vi "游标显示-快关试验.vi"(3 "计算参数 in":T2, 4 "试验模式":string, 5 "reference in":refnum<vi>) -> (0 "计算参数 out":T2, 2 "reference out":refnum<vi>)   [LabVIEW 2013]
panel:
  in  "Array":string[](array[string])=["行程", "电气", "油压1"]
  out "Yrange":dbl
  out "Xrange":dbl
  in  "Cursor":T1
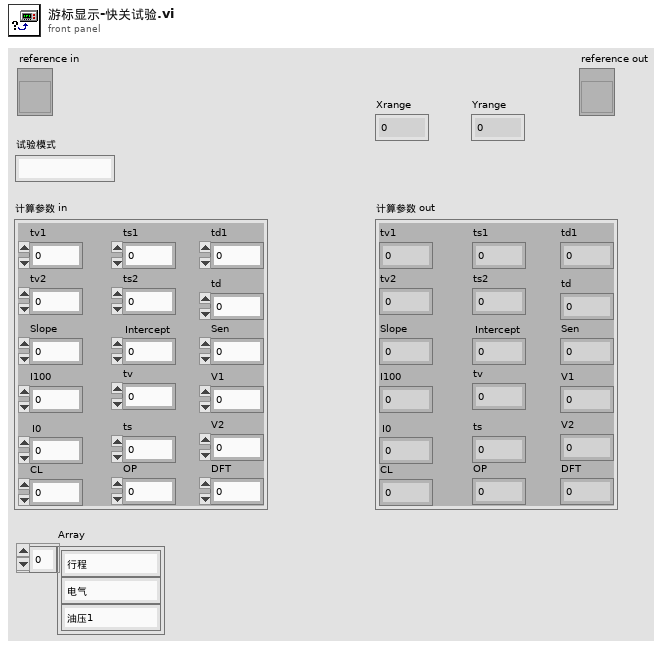
[diagram p1: front panel]
types:
  T1 = cluster{"Name":string, "Color":u32, "Style":u8, "Point Style":u8, "Name Visible":bool, "Allow Drag":bool, "Cursor Mode":u32, "Plot":i32, "Index":i32, "Position":cluster{"X":dbl, "Y":dbl}, "X Scale":u32, "Y Scale":u32, "Watch Plots":i32[], "Watch All Plots":bool, "Plot Area":i32, "Label Offset":cluster{"X":dbl, "Y":dbl}}
  T2 = cluster{"tv1":dbl, "tv2":dbl, "tv":dbl, "ts1":dbl, "ts2":dbl, "ts":dbl, "td1":dbl, "td":dbl, "Slope":dbl, "Intercept":dbl, "I100":dbl, "I0":dbl, "Sen":dbl, "V1":dbl, "V2":dbl, "CL":dbl, "OP":dbl, "DFT":dbl}
  T3 = cluster{"Name":string, "Color":u32, "Style":u8, "Point Style":u8, "Name Visible":bool, "Allow Drag":bool, "Cursor Mode":u32, "Plot":i32, "Index":i32, "Position":cluster{"X":dbl, "Y":dbl}, "X Scale":u32, "Y Scale":u32, "Watch Plots":i32[], "Watch All Plots":bool, "Plot Area":i32, "Label Offset":cluster{"X":dbl, "Y":dbl}}[]
  T4 = typedef "LVCursorListTypeDef.ctl" = cluster{"Name":string, "Color":u32, "Style":u8, "Point Style":u8, "Name Visible":bool, "Allow Drag":bool, "Cursor Mode":u32, "Plot":i32, "Index":i32, "Position":cluster{"X":dbl, "Y":dbl}, "X Scale":u32, "Y Scale":u32, "Watch Plots":i32[], "Watch All Plots":bool, "Plot Area":i32, "Label Offset":cluster{"X":dbl, "Y":dbl}}[]
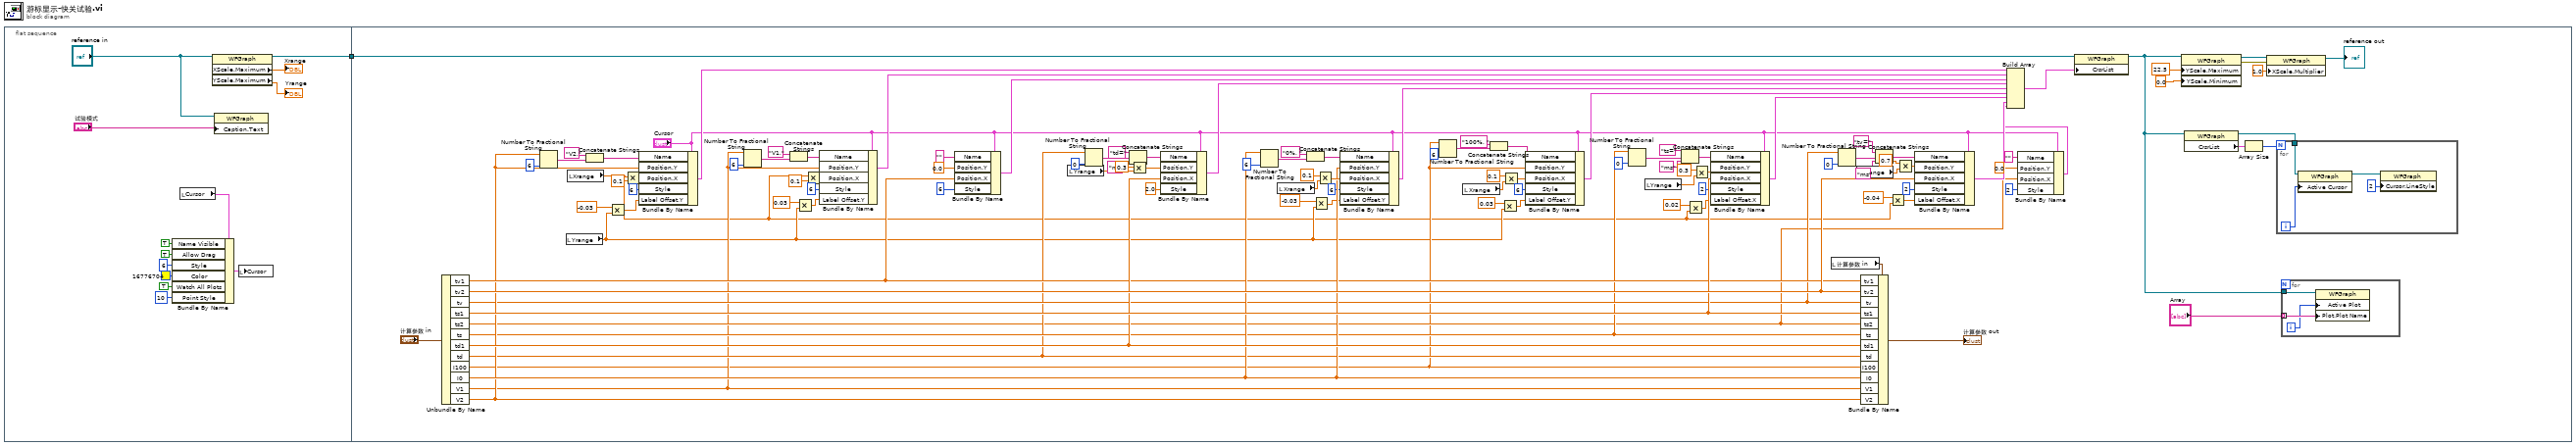
[diagram p0: block diagram]
diagram:
  n1 = flat-sequence {
    tunnel: [w4] -> w1
    tunnel: w1 -> [w44]
    frame #0 {
      n2 = local read "Cursor"() -> (w11:T1)
      n3 = Bundle By Name(cluster=w11, "Name Visible"=TRUE, "Allow Drag"=TRUE, "Style"=u8 6, "Color"=u32 16776704, "Watch All Plots"=TRUE, "Point Style"=u8 10) -> (w10:T1)
      n4 = property class="WFGraph"(reference="reference in") -> (reference out=w4:refnum<vi>, "XScale.Maximum"=→"Xrange":dbl, "YScale.Maximum"=→"Yrange":dbl)  [unwired: 1 in, 1 out]
      n5 = property on="Property Node" class="WFGraph"(reference="reference in", "Caption.Text"="试验模式") -> ()  [unwired: 1 in, 2 out]
      n6 = local write "Cursor"(w10) -> ()
    }
    frame #1 {
      n7 = Unbundle By Name("计算参数 in") -> ("tv1"=w105:dbl, "tv2"=w124:dbl, "tv"=w84:dbl, "ts1"=w120:dbl, "ts2"=w50:dbl, "ts"=w83:dbl, "td1"=w119:dbl, "td"=w52:dbl, "I100"=w35:dbl, "I0"=w111:dbl, "V1"=w48:dbl, "V2"=w96:dbl)
      n8 = Number To Fractional String(number=w96, precision (6)=i16 6 ("宽度(-)")) -> (F-format string=w59:string)  [unwired: 2 in]
      n9 = local read "Yrange"() -> (w25:dbl)
      n10 = local read "Xrange"() -> (w20:dbl)
      n11 = Concatenate Strings("V2," ("光标.游标名"), w59) -> (w95:string)
      n12 = Multiply(x=-0.03 ("y"), y=w25) -> (x*y=w33:dbl)
      n13 = Multiply(x=w20, y=0.1) -> (x*y=w98:dbl)
      n14 = Bundle By Name(cluster="Cursor", "Name"=w95, "Position.Y"=w96, "Position.X"=w98, "Style"=u8 6, "Label Offset.Y"=w33) -> (w87:T1)
      n15 = Number To Fractional String(number=w48, precision (6)=i16 6 ("宽度(-)")) -> (F-format string=w56:string)  [unwired: 2 in]
      n16 = Concatenate Strings("V1," ("光标.游标名"), w56) -> (w49:string)
      n17 = Multiply(x=0.03, y=w25) -> (x*y=w31:dbl)
      n18 = Multiply(x=w20, y=0.1) -> (x*y=w47:dbl)
      n19 = Bundle By Name(cluster="Cursor", "Name"=w49, "Position.Y"=w48, "Position.X"=w47, "Style"=u8 6, "Label Offset.Y"=w31) -> (w46:T1)
      n20 = Bundle By Name(cluster="Cursor", "Name"="", "Position.Y"=0.0, "Position.X"=w105, "Style"=u8 6) -> (w88:T1)
      n21 = local read "Yrange"() -> (w110:dbl)
      n22 = Number To Fractional String(number=w52, precision (6)=i16 0 ("宽度(-)")) -> (F-format string=w76:string)  [unwired: 2 in]
      n23 = Concatenate Strings("td=" ("字符串"), w76, "ms" ("字符串")) -> (w107:string)
      n24 = Multiply(x=0.3 ("y"), y=w110) -> (x*y=w108:dbl)
      n25 = Bundle By Name(cluster="Cursor", "Name"=w107, "Position.Y"=w108, "Position.X"=w119, "Style"=2.0 ("Position.Y")) -> (w89:T1)
      n26 = Number To Fractional String(number=w111, precision (6)=i16 6 ("宽度(-)")) -> (F-format string=w62:string)  [unwired: 2 in]
      n27 = local read "Xrange"() -> (w113:dbl)
      n28 = Concatenate Strings("0%, " ("光标.游标名"), w62) -> (w103:string)
      n29 = Multiply(x=-0.03 ("y"), y=w25) -> (x*y=w28:dbl)
      n30 = Multiply(x=0.1 ("y"), y=w113) -> (x*y=w114:dbl)
      n31 = Bundle By Name(cluster="Cursor", "Name"=w103, "Position.Y"=w111, "Position.X"=w114, "Style"=u8 6, "Label Offset.Y"=w28) -> (w90:T1)
      n32 = Number To Fractional String(number=w35, precision (6)=i16 6 ("宽度(-)")) -> (F-format string=w65:string)  [unwired: 2 in]
      n33 = local read "Xrange"() -> (w117:dbl)
      n34 = Concatenate Strings("100%, " ("光标.游标名"), w65) -> (w102:string)
      n35 = Multiply(x=0.03, y=w25) -> (x*y=w26:dbl)
      n36 = Multiply(x=0.1 ("y"), y=w117) -> (x*y=w116:dbl)
      n37 = Bundle By Name(cluster="Cursor", "Name"=w102, "Position.Y"=w35, "Position.X"=w116, "Style"=u8 6, "Label Offset.Y"=w26) -> (w91:T1)
      n38 = Number To Fractional String(number=w83, precision (6)=i16 0 ("宽度(-)")) -> (F-format string=w77:string)  [unwired: 2 in]
      n39 = local read "Yrange"() -> (w123:dbl)
      n40 = Concatenate Strings("ts=" ("字符串"), w77, "ms" ("字符串")) -> (w104:string)
      n41 = Multiply(x=0.02, y=w20) -> (x*y=w23:dbl)
      n42 = Multiply(x=0.3 ("y"), y=w123) -> (x*y=w122:dbl)
      n43 = Bundle By Name(cluster="Cursor", "Name"=w104, "Position.Y"=w122, "Position.X"=w120, "Style"=u8 2, "Label Offset.X"=w23) -> (w92:T1)
      n44 = local read "计算参数 in"() -> (w82:T2)
      n45 = Number To Fractional String(number=w84, precision (6)=i16 0 ("宽度(-)")) -> (F-format string=w70:string)  [unwired: 2 in]
      n46 = local read "Yrange"() -> (w127:dbl)
      n47 = Bundle By Name(cluster=w82, "tv1"=w105, "tv2"=w124, "tv"=w84, "ts1"=w120, "ts2"=w50, "ts"=w83, "td1"=w119, "td"=w52, "I100"=w35, "I0"=w111, "V1"=w48, "V2"=w96) -> (→"计算参数 out":T2)
      n48 = Concatenate Strings("tv=" ("字符串"), w70, "ms" ("字符串")) -> (w118:string)
      n49 = Multiply(x=-0.04, y=w20) -> (x*y=w21:dbl)
      n50 = Multiply(x=0.7 ("y"), y=w127) -> (x*y=w126:dbl)
      n51 = Bundle By Name(cluster="Cursor", "Name"=w118, "Position.Y"=w126, "Position.X"=w124, "Style"=u8 2, "Label Offset.X"=w21) -> (w93:T1)
      n52 = Bundle By Name(cluster="Cursor", "Name"="", "Position.Y"=0.0, "Position.X"=w50, "Style"=u8 2) -> (w51:T1)
      n53 = Build Array(w87, w46, w88, w89, w90, w91, w92, w93, w51) -> (w94:T3)
      n54 = property class="WFGraph"(reference=w44, "CrsrList"=w94) -> (reference out=w15:refnum<vi>)  [unwired: 1 in, 1 out]
      n55 = property on="属性节点" class="WFGraph"(reference=w15, "YScale.Maximum"=22.5 ("Y标尺.范围:最大值"), "YScale.Minimum"=0.0 ("Y标尺.范围:最小值")) -> (reference out=w100:refnum<vi>, error out=w101:errorcluster)  [unwired: 1 in]
      n56 = property class="WFGraph"(reference=w15) -> (reference out=w17:refnum<vi>, "CrsrList"=w19:T4)  [unwired: 1 in, 1 out]
      n57 = Array Size(array=w19) -> (size(s)=w18:i32)
      n58 = property on="属性节点" class="WFGraph"(reference=w100, error in=w101, "XScale.Multiplier"=1.0 ("X标尺.偏移量与缩放系数:缩放系数")) -> (reference out=→"reference out":refnum<vi>)  [unwired: 1 out]
      n59 = for {
        N: w18 -> [_]
        tunnel: w17 -> [w136]
        i -> [w135]
        n60 = property class="WFGraph"(reference=w136, "Active Cursor"=w135) -> (reference out=w134:refnum<vi>)  [unwired: 1 in, 1 out]
        n61 = property class="WFGraph"(reference=w134, "Cursor.LineStyle"=u8 2 ("Cursor.Line Style")) -> ()  [unwired: 1 in, 2 out]
      }
      n62 = for {
        tunnel: "Array" -> [w132] mode=indexing
        tunnel: w15 -> [w131]
        i -> [w130]
        n63 = property class="WFGraph"(reference=w131, "Active Plot"=w130, "Plot.Plot Name"=w132) -> ()  [unwired: 1 in, 2 out]
      }
    }
  }
